vi "MainNR.vi"(10 "JQMHStartup":refnum<class "RQMHStartup.lvclass">, 11 "TemplateModule in":refnum<class "TemplateModule.lvclass">) -> ()   [LabVIEW 2024, in "TemplateModule.lvclass"]
uses:
  TemplateModule.lvclass
  RQMHCore/Startup/RQMHStartup.lvclass
  RQMHCore/ModQueue/RQMHMessageQueue.lvclass/RQMHMessageQueue.ctl
  RQMHCore/ModuleCore/InitialiseReplyArgs.ctl
  <vilib>/Utility/miscctls.llb/LVPointTypeDef.ctl
  RQMHCore/ModuleCore/RQMHModule.lvclass/RQMHModule.ctl
  Do Something ReplyArgs.ctl
  Do Something Args.ctl
  JamesT ReplyArgs.ctl
  JamesT Args.ctl
  test Args.ctl
  testering Args.ctl
  RQMHCore/ModuleCore/RQMHModule.lvclass
  RQMHCore/ModuleCore/Read ModuleName.vi
  RQMHCore/ModuleCore/Read External Start.vi
  RQMHCore/ModQueue/Delacor_lib_QMH_Enqueue Message (Single).vi
  RQMHCore/ModQueue/RQMHMessageQueue.lvclass
  TemplateModule.lvclass/TemplateModule.ctl
  RQMHCore/Shared/RQMHShared.lvlib
panel:
  out "error out":errorcluster
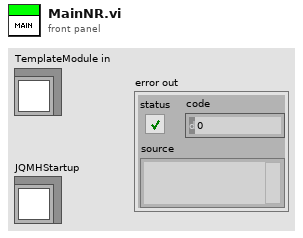
[diagram p1: front panel]
types:
  T1 = typedef "TemplateModule.lvclass/Request Events--cluster.ctl" = cluster{"Do Something":refnum<user-event>, "JamesT":refnum<user-event>, "RRRR":refnum<user-event>, refnum<user-event>, "test":refnum<user-event>, "testering":refnum<user-event>}
  T2 = cluster{"Stop Module":refnum<user-event>, "Requests":T1}
  T3 = typedef "LVPointTypeDef.ctl" = cluster{"Horizontal":i16, "Vertical":i16}
  T4 = enum32{"Invalid", "Standard", "Closed", "Hidden", "Minimized", "Maximized"}
  T5 = typedef "RQMHModule.lvclass/InitialiseReplyArgs.ctl" = cluster{"Did Init?":bool}
  T6 = typedef "TemplateModule.lvclass/Do Something Args.ctl" = cluster{"Msg":string}
  T7 = typedef "TemplateModule.lvclass/Do Something ReplyArgs.ctl" = cluster{"Value":dbl, "Boolean":bool}
  T8 = typedef "TemplateModule.lvclass/JamesT Args.ctl" = cluster{"Boolean":bool}
  T9 = typedef "TemplateModule.lvclass/JamesT ReplyArgs.ctl" = cluster{"String":string}
  T10 = typedef "TemplateModule.lvclass/test Args.ctl" = cluster{"String":string}
  T11 = typedef "TemplateModule.lvclass/testering Args.ctl" = cluster{"RQMHModule.lvclass":refnum<class "RQMHModule.lvclass">}
  T12 = typedef "RQMHModule.lvclass/Reply.ctl" = cluster{"Expects Reply":bool, "Reply":refnum<notifier>}
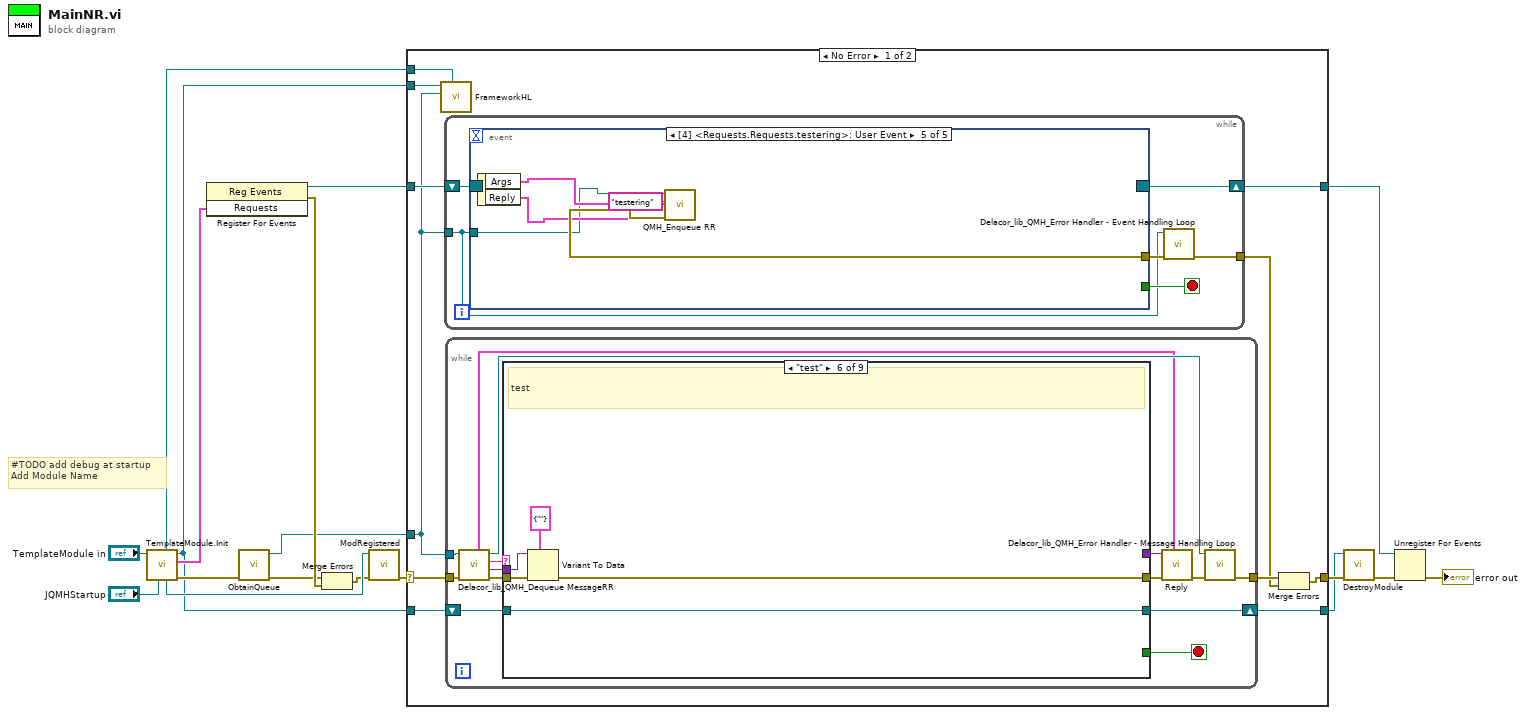
[diagram p0: block diagram]
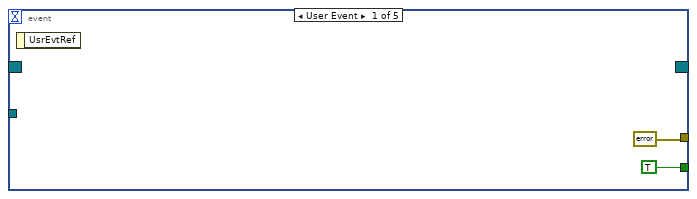
[diagram p2: hidden frame]
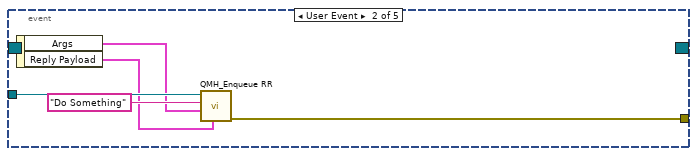
[diagram p3: hidden frame]
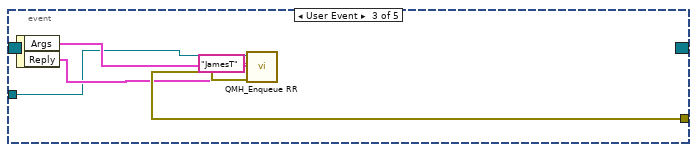
[diagram p4: hidden frame]
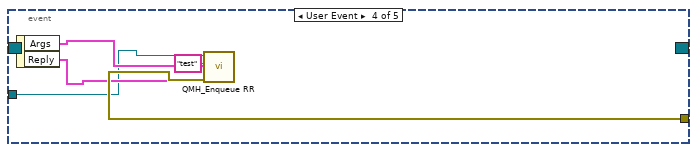
[diagram p5: hidden frame]
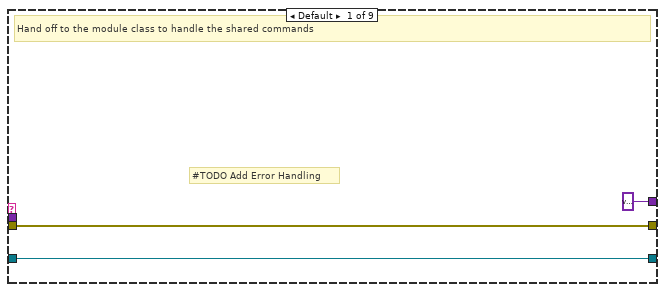
[diagram p6: hidden frame]
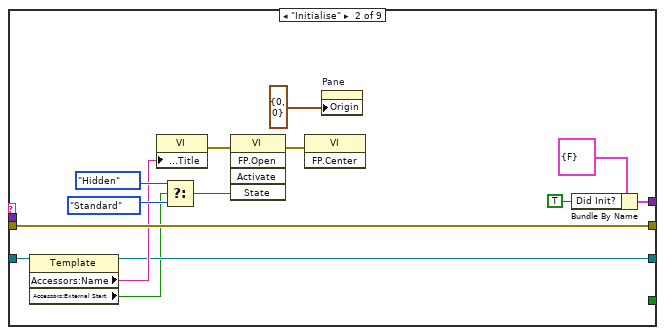
[diagram p7: hidden frame]
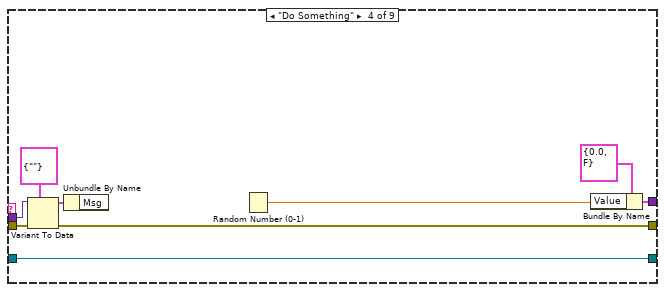
[diagram p9: hidden frame]
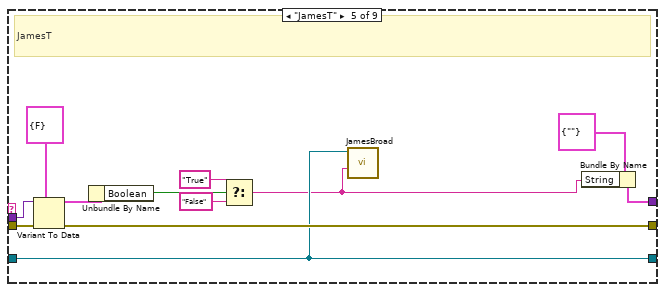
[diagram p10: hidden frame]
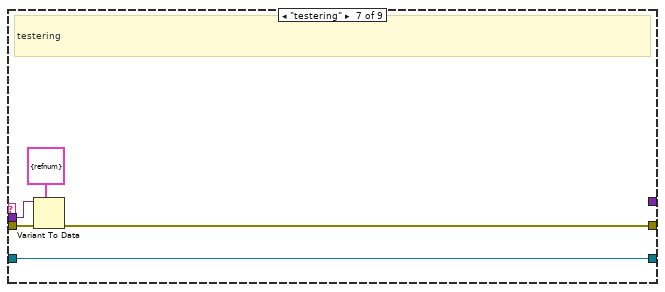
[diagram p11: hidden frame]
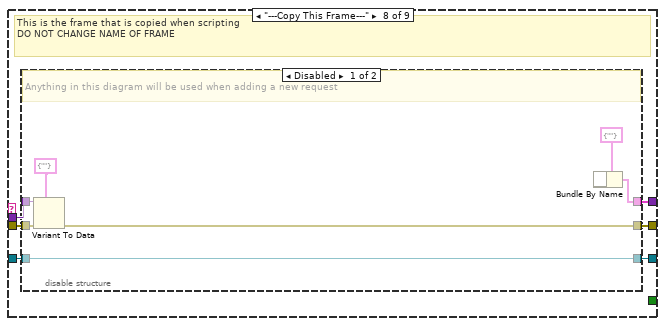
[diagram p12: hidden frame]
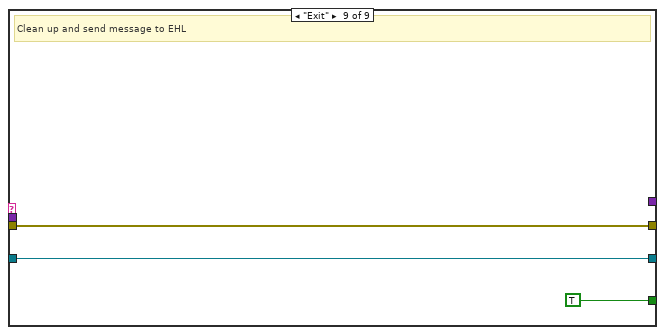
[diagram p14: hidden frame]
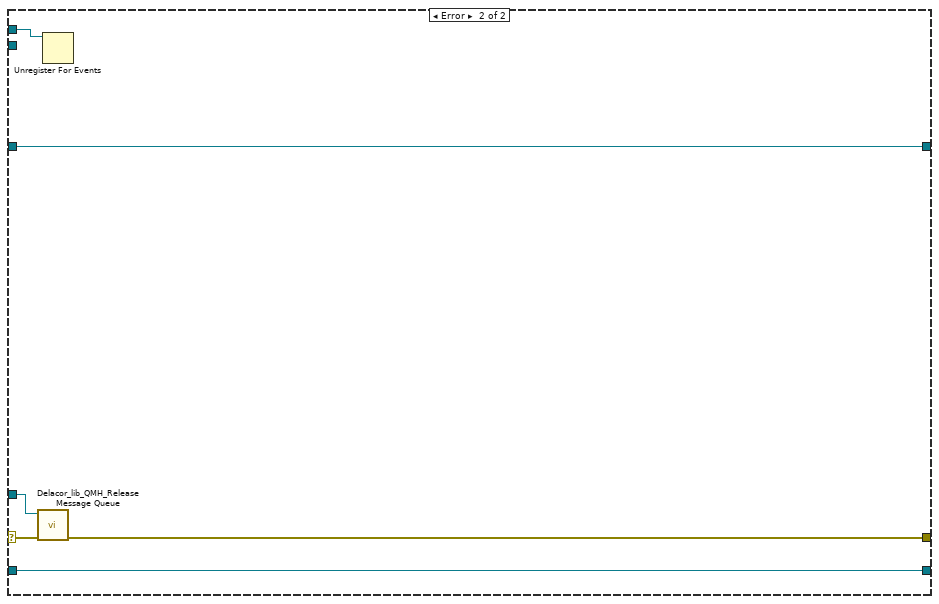
[diagram p15: hidden frame]
diagram:
  # "#TODO add debug at startup\nAdd Module Name"
  n1 = call "TemplateModule.Init.vi"("JQMHStartup in"="JQMHStartup", "TemplateModule in"="TemplateModule in") -> ("error out"=w11:errorcluster, "Requests"=w2:T2, "TemplateModule out"=w1:refnum<class "TemplateModule.lvclass">, "JQMHStartup out"=w9:refnum<class "RQMHStartup.lvclass">, "StandardRequests"=w5:refnum<event-registration>)  [unwired: 4 in, 1 out]
  n2 = register-events(w2) -> (reference out=w4:refnum<event-registration>, error out=w18:errorcluster)  [unwired: 2 in]
  n3 = call "ObtainQueue.vi"("error in"=w11) -> ("error out"=w10:errorcluster, "Message Queue"=w6:refnum<class "RQMHMessageQueue.lvclass">)  [unwired: 9 in]
  n4 = Merge Errors(w10, w18) -> (w7:errorcluster)
  n5 = call "ModRegistered.vi"("error in (no error)"=w7, "JQMHStartup in"=w9) -> ("error out"=w8:errorcluster)  [unwired: 9 in]
  n6 = case "RQMH_MAIN" shown="No Error" w8 {
    selector: w8 -> [w26 w143]
    tunnel: w1 -> [w29 w142]
    tunnel: [w28 w145] -> w17
    tunnel: w4 -> [w27 w145]
    tunnel: w6 -> [w20 w144]
    tunnel: [w25 w142] -> w3
    tunnel: [w22 w141] -> w14
    tunnel: w1 -> [w21 _]
    tunnel: w5 -> [w19 w140]
    frame No Error {
      n7 = call-dynamic "FrameworkHL.vi"("StandardRequests"=w19, "Message Queue"=w20, "JQMHModule in"=w21) -> ()  [unwired: 9 in]
      n8 = while {
        shift-right: [w35] -> w28
        shift-left: w27 -> [w30]
        tunnel: w20 -> [w31]
        tunnel: [w32] -> w23
        stop <- w34 stop-if-true
        n9 = event "RQMH_EVENT_MAIN" shown="[4] <Requests.Requests.testering>: User Event" {
          selector: w30 -> [_ _ _ _ _]
          dyn-events: [_ _ _ _ _] -> w35
          timeout: _ -> [_ _ _ _ _]
          tunnel: [TRUE _ _ _ _] -> w34
          tunnel: w31 -> [_ w42 w44 w49 w54]
          tunnel: [errorcluster {"status"=FALSE, "code"=0, "source"=""} ("error out") w39 w47 w52 w57] -> w33
          event User Event {
            n10 = event-data() -> ()  [unwired: 1 in, 1 out]
          }
          event User Event {
            n11 = event-data() -> ("Args"=w40:T6, "Reply Payload"=w38:T12)  [unwired: 1 in]
            n12 = call "QMH_Enqueue RR.vi"("Reply"=w38, "Message Data"=w40, "Message"="Do Something", "Message Queue in"=w42) -> ("error out"=w39:errorcluster)  [unwired: 6 in, 1 out]
          }
          event User Event {
            n13 = event-data() -> ("Args"=w45:T8, "Reply"=w46:T12)  [unwired: 1 in]
            n14 = call "QMH_Enqueue RR.vi"("Reply"=w46, "Message Data"=w45, "Message"="JamesT", "Message Queue in"=w44) -> ("error out"=w47:errorcluster)  [unwired: 6 in, 1 out]
          }
          event User Event {
            n15 = event-data() -> ("Args"=w50:T10, "Reply"=w51:T12)  [unwired: 1 in]
            n16 = call "QMH_Enqueue RR.vi"("Reply"=w51, "Message Data"=w50, "Message"="test", "Message Queue in"=w49) -> ("error out"=w52:errorcluster)  [unwired: 6 in, 1 out]
          }
          event User Event {
            n17 = event-data() -> ("Args"=w55:T11, "Reply"=w56:T12)  [unwired: 1 in]
            n18 = call "QMH_Enqueue RR.vi"("Reply"=w56, "Message Data"=w55, "Message"="testering", "Message Queue in"=w54) -> ("error out"=w57:errorcluster)  [unwired: 6 in, 1 out]
          }
        }
        n19 = call-dynamic "Delacor_lib_QMH_Error Handler - Event Handling Loop.vi"("error in"=w33, "Message Queue in"=w31) -> ("dup error in"=w32:errorcluster)  [unwired: 8 in, 1 out]
      }
      n20 = while {
        tunnel: w20 -> [w66]
        tunnel: w26 -> [w65]
        shift-right: [w68] -> w25
        shift-left: w29 -> [w69]
        tunnel: [w67] -> w24
        stop <- w71 stop-if-true
        n21 = call-dynamic "Delacor_lib_QMH_Dequeue MessageRR.vi"("error in"=w65, "Message Queue in"=w66) -> ("error out"=w64:errorcluster, "Message Data"=w62:variant, "Message"=w63:string, "Message Queue out"=w70:refnum<class "RQMHMessageQueue.lvclass">, "Reply"=w58:T12)  [unwired: 5 in]
        n22 = case "RQMH_MESSAGE_CASES" shown="\"test\"" w63 {
          tunnel: [_ _ _ _ _ _ _ _ TRUE] -> w71
          tunnel: w69 -> [w73 w76 w89 w99 w107 w114 w119 w125 w138]
          tunnel: w62 -> [_ _ _ w95 w109 w113 w118 w123 _]
          tunnel: w64 -> [w74 w88 w90 w94 w111 w116 w121 w127 w137]
          tunnel: [w74 w88 w90 w93 w110 w115 w120 w126 w137] -> w61
          tunnel: [w73 w77 w89 w99 w107 w114 w119 w124 w138] -> w68
          tunnel: [variant w87 _ w98 w108 _ _ w122 _] -> w59
          frame Default {
            # "#TODO Add Error Handling"
            # "Hand off to the module class to handle the shared commands"
          }
          frame "Initialise" {
            n23 = property class="Template"(reference=w76) -> (reference out=w77:refnum<class "TemplateModule.lvclass">, "Accessors:Name"=w78:string, "Accessors:External Start"=w75:bool)  [unwired: 1 in, 1 out]
            n24 = property on="Property Node" class="VI"("Front Panel.Title"=w78) -> (error out=w85:errorcluster)  [unwired: 2 in, 1 out]
            n25 = Select(t=T4."Hidden" ("State"), s=w75, f=T4."Standard" ("State")) -> (s? t:f=w81:T4)
            n26 = invoke on="Invoke Node" class="VI" method="FP.Open"(error in=w85, "State"=w81) -> (error out=w84:errorcluster)  [unwired: 3 in, 4 out]
            n27 = invoke on="Invoke Node" class="VI" method="FP.Center"(error in=w84) -> ()  [unwired: 2 in, 3 out]
            n28 = property on="Pane" class="Pane"("Origin"=T3 {"Horizontal"=0, "Vertical"=0}) -> ()  [unwired: 2 in, 2 out]
            n29 = Bundle By Name(cluster=T5 {"Did Init?"=FALSE} ("Args"), "Did Init?"=TRUE) -> (w87:T5)
          }
          frame "---Module Specific---" {
          }
          frame "Do Something" {
            n30 = Variant To Data(error in=w94, type=T6 {"Msg"=""} ("Do Something Args"), Variant=w95) -> (data=w91:T6, error out=w93:errorcluster)
            n31 = Unbundle By Name(w91) -> ()  [unwired: 1 out]
            n32 = Random Number (0-1)() -> (number: 0 to 1=w96:dbl)
            n33 = Bundle By Name(cluster=T7 {"Value"=0.0, "Boolean"=FALSE}, "Value"=w96) -> (w98:T7)
          }
          frame "JamesT" {
            # "JamesT"
            n34 = Variant To Data(error in=w111, type=T8 {"Boolean"=FALSE} ("Args"), Variant=w109) -> (data=w106:T8, error out=w110:errorcluster)
            n35 = Unbundle By Name(w106) -> ("Boolean"=w105:bool)
            n36 = Select(t="True", s=w105, f="False") -> (s? t:f=w101:string)
            n37 = call "JamesBroad.vi"("String"=w101, "TemplateModule in"=w107) -> ()  [unwired: 8 in, 2 out]
            n38 = Bundle By Name(cluster=T9 {"String"=""} ("RQMH_MHL_REPLY_PL"), "String"=w101) -> (w108:T9)
          }
          frame "test" {
            # "test"
            n39 = Variant To Data(error in=w116, type=T10 {"String"=""} ("RQMH_MHL_MSG_PL"), Variant=w113) -> (error out=w115:errorcluster)  [unwired: 1 out]
          }
          frame "testering" {
            # "testering"
            n40 = Variant To Data(error in=w121, type=T11 {"RQMHModule.lvclass"=refnum} ("RQMH_MHL_MSG_PL"), Variant=w118) -> (error out=w120:errorcluster)  [unwired: 1 out]
          }
          frame "---Copy This Frame---" {
            # "This is the frame that is copied when scripting\nDO NOT CHANGE NAME OF FRAME"
            n41 = disable-structure shown="Disabled" {
              disable-tunnel: w127 -> [w131 w136]
              disable-tunnel: [w132 w136] -> w126
              disable-tunnel: w125 -> [w134 w135]
              disable-tunnel: [w134 w135] -> w124
              disable-tunnel: w123 -> [w133 _]
              disable-tunnel: [w129 _] -> w122
              frame Disabled {
                # "Anything in this diagram will be used when adding a new request"
                n42 = Variant To Data(error in=w131, type=cluster{string} {""} ("RQMH_MHL_MSG_PL"), Variant=w133) -> (error out=w132:errorcluster)  [unwired: 1 out]
                n43 = Bundle By Name(cluster=cluster{string} {""} ("RQMH_MHL_REPLY_PL")) -> (w129:cluster{string})  [unwired: 1 in]
              }
              frame Enabled {
              }
            }
          }
          frame "Exit" {
            # "Clean up and send message to EHL"
          }
        }
        n44 = call "Reply.vi"("Reply"=w58, "error in (no error)"=w61, "ReplyPayload"=w59) -> ("error out"=w60:errorcluster)  [unwired: 8 in]
        n45 = call-dynamic "Delacor_lib_QMH_Error Handler - Message Handling Loop.vi"("error in"=w60, "Message Queue in"=w70) -> ("dup error in"=w67:errorcluster)  [unwired: 8 in, 1 out]
      }
      n46 = Merge Errors(w24, w23) -> (w22:errorcluster)
    }
    frame Error {
      n47 = call-dynamic "Delacor_lib_QMH_Release Message Queue.vi"("error in"=w143, "Message Queue"=w144) -> ("error out"=w141:errorcluster)  [unwired: 9 in]
      n48 = Unregister For Events(event registration refnum=w140) -> ()  [unwired: 1 in, 1 out]
    }
  }
  n49 = call "DestroyModule.vi"("error in (no error)"=w14, "JQMHModule in"=w3) -> ("error out"=w16:errorcluster)  [unwired: 9 in]
  n50 = Unregister For Events(event registration refnum=w17, error in=w16) -> (error out=→"error out":errorcluster)
